vi "SetAdapTorrMode_v0.vi"(2 "Debug Mode":bool, 3 "Elapsed Time (s)":dbl, 4 "State":enum16{"Edit", "Start", "Run", "End", "Idle"}(ring), 5 "Argument List In":string[](array[string])) -> (0 "Status Out":string, 1 "Argument List Out":string[](array[string]))   [LabVIEW 2011]
panel:
  in  "Mode":u16(ring) items=["Setpoint A (Remote)", "Setpoint B (Remote)", "Setpoint C (Remote)", "Setpoint D  (Remote)", "Open (Remote)", "Close (Remote)", "Hold (Remote)", "Hold (Local)"]
  in  "error in (no error)":errorcluster
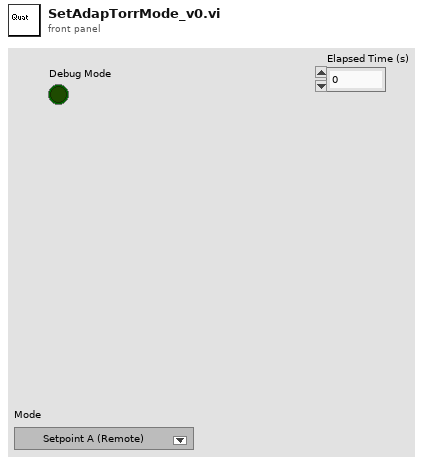
[diagram p1: front panel]
types:
  T1 = enum32{"Invalid", "Default", "Floating", "Floating/Auto-Hide", "Modal"}
  T2 = enum16{"Discrete", "Continuous", "Instantaneous"}
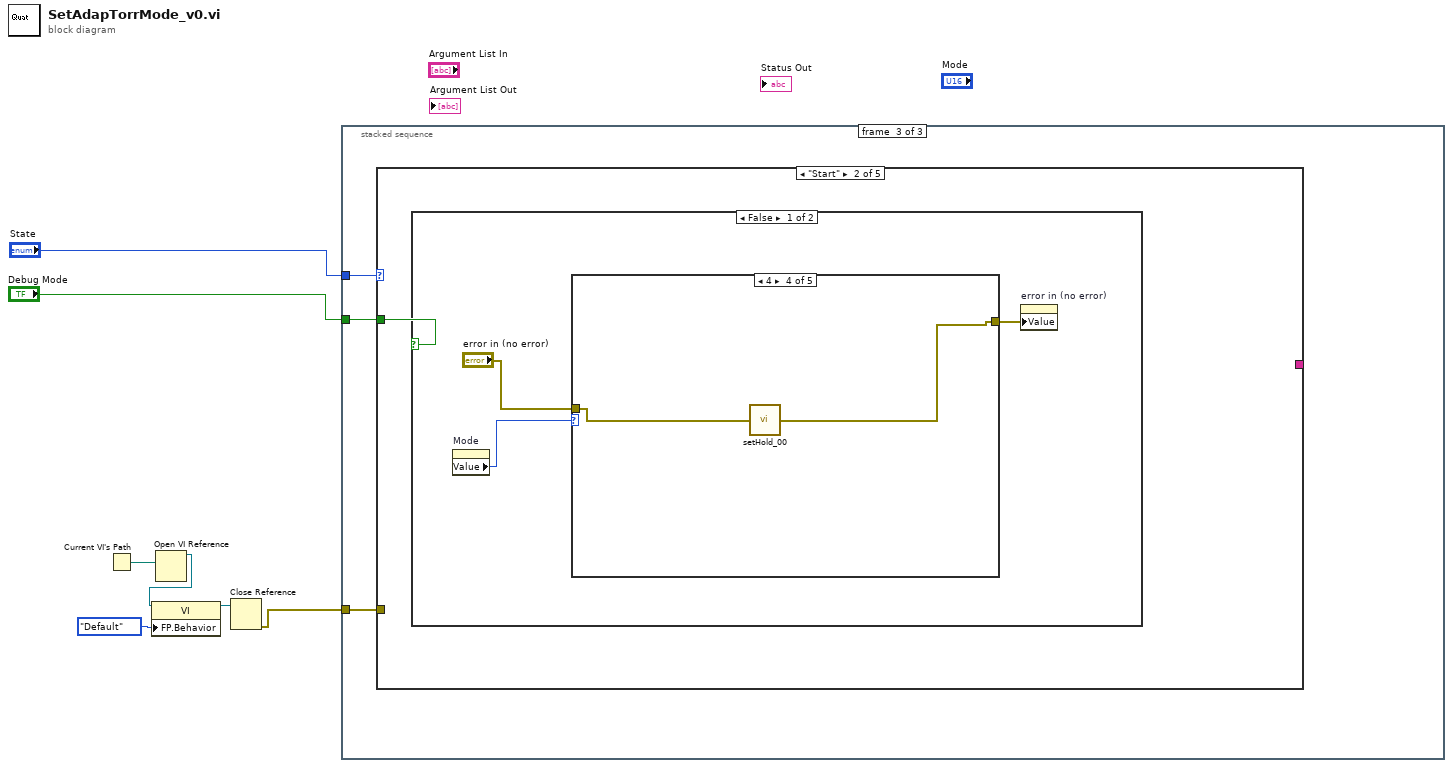
[diagram p0: block diagram]
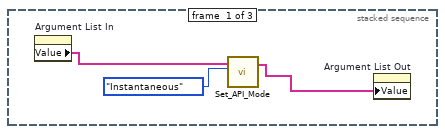
[diagram p2: hidden frame]
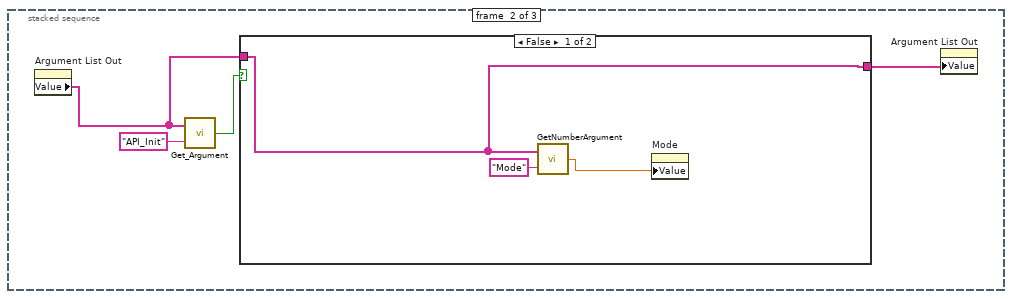
[diagram p3: hidden frame]
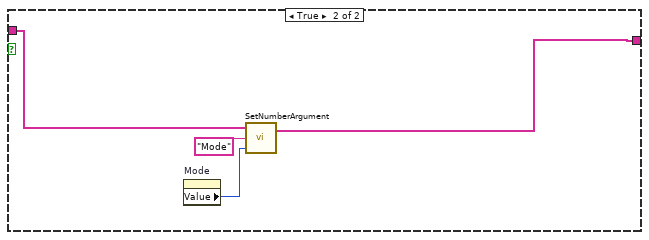
[diagram p4: hidden frame]
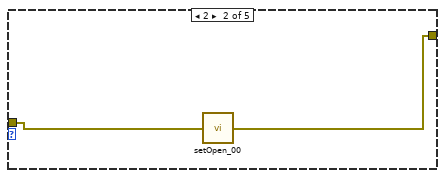
[diagram p7: hidden frame]
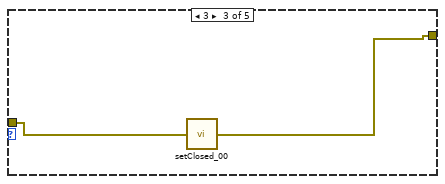
[diagram p8: hidden frame]
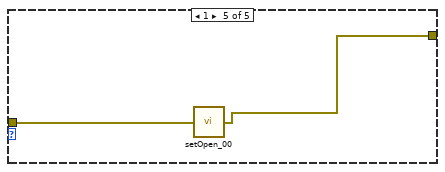
[diagram p9: hidden frame]
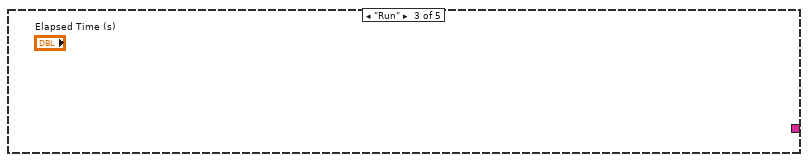
[diagram p11: hidden frame]
diagram:
  n1 = Current VI's Path() -> (path=w5:path)
  n2 = Open VI Reference(vi path=w5) -> (vi reference=w4:refnum<vi>)  [unwired: 1 in, 5 out]
  n3 = property class="VI"(reference=w4, "FP.Behavior"=T1."Default" ("Front Panel Window:Behavior")) -> (reference out=w2:refnum<vi>)  [unwired: 1 in, 1 out]
  n4 = Close Reference(reference=w2) -> (error out=w1:errorcluster)  [unwired: 1 in]
  n5 = stacked-sequence {
    tunnel: "State" -> [_ _ w24]
    tunnel: "Debug Mode" -> [_ _ w23]
    tunnel: w1 -> [_ _ w22]
    frame #0 {
      n6 = property on="Argument List In" class="Arr (strict)"() -> ("Value"=w9:string[])  [unwired: 2 in, 2 out]
      n7 = call "Set_API_Mode.vi"("API Mode"=T2."Instantaneous", "Argument List In"=w9) -> ("Argument List Out"=w8:string[])  [unwired: 3 in]
      n8 = property on="Argument List Out" class="Arr (strict)"("Value"=w8) -> ()  [unwired: 2 in, 2 out]
    }
    frame #1 {
      n9 = property on="Argument List Out" class="Arr (strict)"() -> ("Value"=w12:string[])  [unwired: 2 in, 2 out]
      n10 = call "Get_Argument.vi"("Argument"="API_Init", "Argument List"=w12) -> ("Enabled"=w13:bool)
      n11 = case shown="False" w13 {
        tunnel: w12 -> [w17 w19]
        tunnel: [w17 w18] -> w11
        frame False {
          n12 = call "GetNumberArgument.vi"("Argument"="Mode", "Argument List In"=w17) -> ("value"=w16:dbl)
          n13 = property on="Mode" class="Ring (strict)"("Value"=w16) -> ()  [unwired: 2 in, 2 out]
        }
        frame True {
          n14 = property on="Mode" class="Ring (strict)"() -> ("Value"=w20:u16)  [unwired: 2 in, 2 out]
          n15 = call "SetNumberArgument.vi"("value"=w20, "Argument"="Mode", "Argument List In"=w19) -> ("Argument List Out"=w18:string[])  [unwired: 1 out]
        }
      }
      n16 = property on="Argument List Out" class="Arr (strict)"("Value"=w11) -> ()  [unwired: 2 in, 2 out]
    }
    frame #2 {
      n17 = case shown="\"Start\"" w24 {
        tunnel: _ -> [w25 _ w38 w39 w40]
        tunnel: w23 -> [_ w26 _ _ _]
        tunnel: w22 -> [_ _ _ _ _]
        frame "Edit", Default {
        }
        frame "Start" {
          n18 = case shown="False" w26 {
            frame False {
              n19 = property on="Mode" class="Ring (strict)"() -> ("Value"=w27:u16)  [unwired: 2 in, 2 out]
              n20 = case shown="4" w27 {
                tunnel: "error in (no error)" -> [_ w31 w33 w35 w37]
                tunnel: [_ w30 w32 w34 w36] -> w28
                frame 0, Default {
                }
                frame 2 {
                  n21 = call "setOpen_00.vi"("error in (no error)"=w31) -> ("error out"=w30:errorcluster)
                }
                frame 3 {
                  n22 = call "setClosed_00.vi"("error in (no error)"=w33) -> ("error out"=w32:errorcluster)
                }
                frame 4 {
                  n23 = call "setHold_00.vi"("error in (no error)"=w35) -> ("error out"=w34:errorcluster)
                }
                frame 1 {
                  n24 = call "setOpen_00.vi"("error in (no error)"=w37) -> ("error out"=w36:errorcluster)
                }
              }
              n25 = property on="error in (no error)" class="Clust (strict)"("Value"=w28) -> ()  [unwired: 2 in, 2 out]
            }
            frame True {
            }
          }
        }
        frame "Run" {
        }
        frame "End" {
        }
        frame "Idle" {
        }
      }
    }
  }
